vi "subStage_ReadExcelToTable.vi"(8 "error in (no error)":errorcluster, 11 "File Path":path) -> (0 "error out":errorcluster, 3 "Record Table":string[][](table))   [LabVIEW 2015]
panel:
  in  "Excel._Application":refnum<k7>
  in  "Excel._Worksheet":refnum<k7>
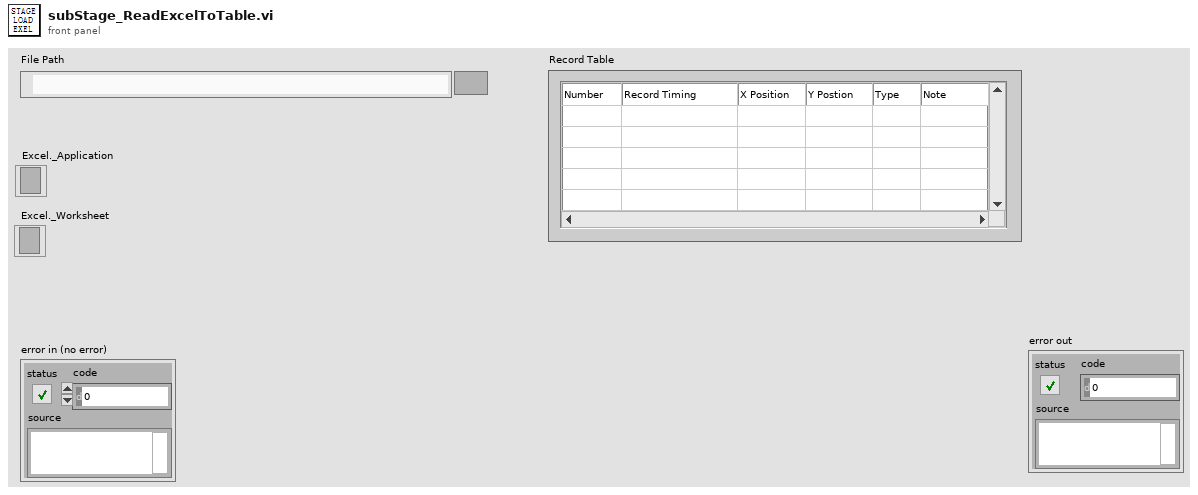
[diagram p1: front panel]
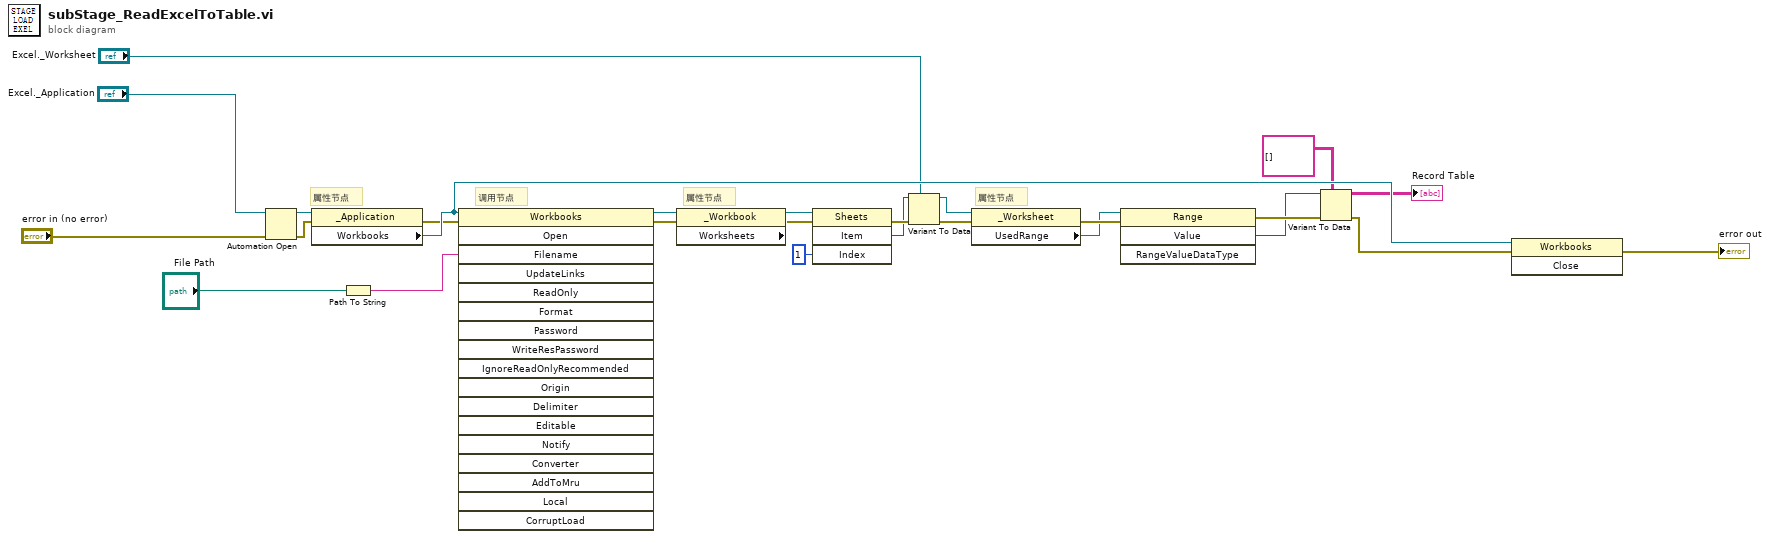
[diagram p0: block diagram]
diagram:
  # "属性节点"
  # "属性节点"
  # "属性节点"
  # "调用节点"
  n1 = Automation Open(error in (no error)="error in (no error)", Automation Refnum="Excel._Application") -> (Automation Refnum=w6:refnum<k7>, error out=w2:errorcluster)  [unwired: 2 in]
  n2 = property class="_Application"(reference=w6, error in=w2) -> (error out=w7:errorcluster, "Workbooks"=w26:refnum<k7>)  [unwired: 1 out]
  n3 = Path To String(path="File Path") -> (string=w23:string)
  n4 = invoke class="Workbooks" method="Open"(reference=w26, error in=w7, "Filename"=w23) -> (error out=w10:errorcluster, "Open"=w9:refnum<k7>)  [unwired: 15 in, 16 out]
  n5 = property class="_Workbook"(reference=w9, error in=w10) -> (error out=w11:errorcluster, "Worksheets"=w25:refnum<k7>)  [unwired: 1 out]
  n6 = invoke class="Sheets" method="Item"(reference=w25, error in=w11, "Index"=1) -> (error out=w13:errorcluster, "Item"=w12:variant)  [unwired: 1 in, 2 out]
  n7 = Variant To Data(error in=w13, type="Excel._Worksheet", Variant=w12) -> (data=w14:refnum<k7>, error out=w15:errorcluster)
  n8 = property class="_Worksheet"(reference=w14, error in=w15) -> (error out=w17:errorcluster, "UsedRange"=w16:refnum<k7>)  [unwired: 1 out]
  n9 = invoke class="Range" method="Value"(reference=w16, error in=w17) -> (error out=w19:errorcluster, "Value"=w18:variant)  [unwired: 2 in, 2 out]
  n10 = Variant To Data(error in=w19, type=string[][] [], Variant=w18) -> (data=→"Record Table":string[][], error out=w24:errorcluster)
  n11 = invoke class="Workbooks" method="Close"(reference=w26, error in=w24) -> (error out=→"error out":errorcluster)  [unwired: 1 in, 2 out]
